vi "Sp To Type.vi"(0 "SP DUT":dbl) -> (4 "Sp_type":T1)   [LabVIEW 2019, in "Stand.lvclass"]
uses:
  Stand.lvclass
  TypeDef/SP_TYPE.ctl
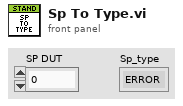
[diagram p1: front panel]
types:
  T1 = typedef "SP_TYPE.ctl" = enum16{"ERROR", "ZIRO", "BASE", "SP"}
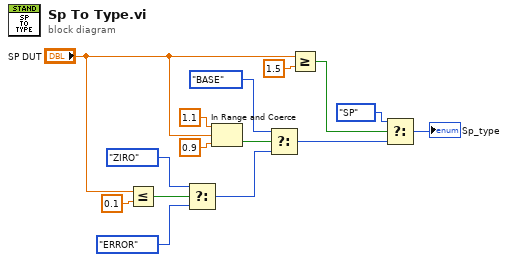
[diagram p0: block diagram]
diagram:
  n1 = Less Or Equal?(x="SP DUT", y=0.1) -> (x <= y?=w13:bool)
  n2 = Select(t=SP_TYPE."ZIRO", s=w13, f=SP_TYPE."ERROR" ("Data.SP_TYPE_DUT")) -> (s? t:f=w11:T1)
  n3 = In Range and Coerce(upper limit=1.1, x="SP DUT", lower limit=0.9) -> (In Range?=w7:bool)  [unwired: 1 out]
  n4 = Select(t=SP_TYPE."BASE", s=w7, f=w11) -> (s? t:f=w6:T1)
  n5 = Greater Or Equal?(x="SP DUT", y=1.5 ("x")) -> (x >= y?=w3:bool)
  n6 = Select(t=SP_TYPE."SP", s=w3, f=w6) -> (s? t:f=→"Sp_type":T1)
